vi "Pfeiffer-RVC300.ProcEvents.vi"(0 "i ref in":refnum<vi>, 5 "error in":errorcluster) -> (14 "i ref out":refnum<vi>, 19 "error out":errorcluster)   [LabVIEW 2014, in "Pfeiffer-RVC300.lvlib"]
doc: "This method is used to define the events the object will listen to. Add your own events here."
uses:
  Pfeiffer-RVC300.lvlib
  CS_Core/BaseProcess/BaseProcess.event definition.ctl
  CS_Core/CAEObj/CAEObj.event definition.ctl
  CS_Core/BaseProcess/BaseProcess.descriptor string definition.ctl
  CS_Core/BaseProcess/BaseProcess.lvlib
  CS_Core/CAEObj/CAEObj.lvlib
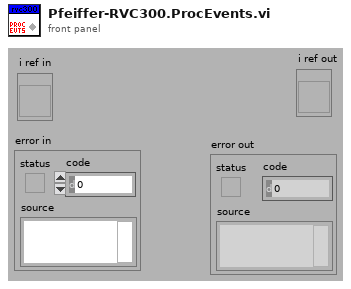
[diagram p1: front panel]
types:
  T1 = typedef "BaseProcess.lvlib/BaseProcess.event definition.ctl" = cluster{"CAEEvtDef":T2, "Data Descriptor":T3}
  T2 = typedef "CAEObj.lvlib/CAEObj.event definition.ctl" = cluster{"URL":string, "enable":bool, "ignoreResID":bool}
  T3 = typedef "BaseProcess.lvlib/BaseProcess.descriptor string definition.ctl" = string
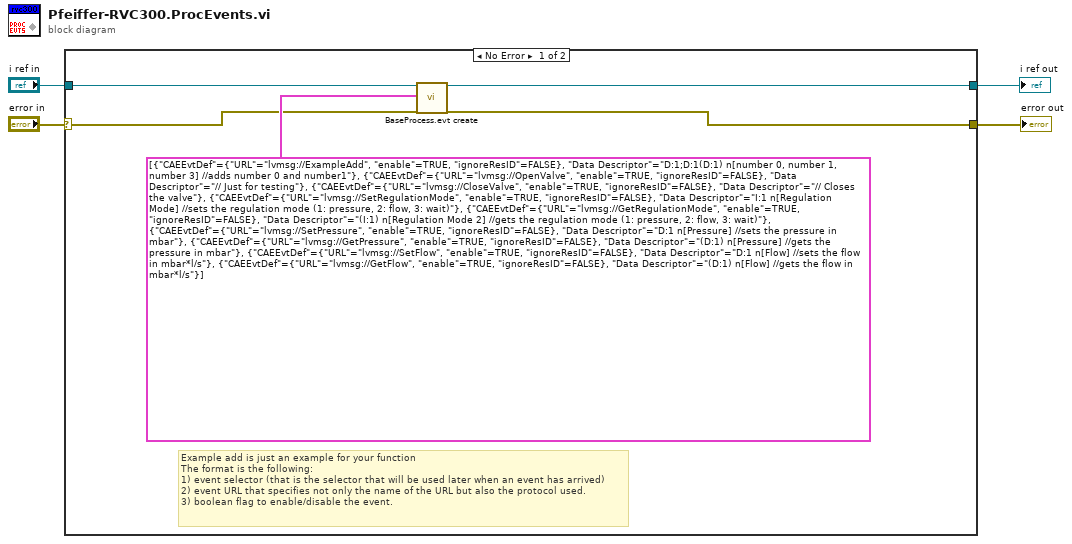
[diagram p0: block diagram]
diagram:
  n1 = case shown="No Error" "error in" {
    selector: "error in" -> [w5 w10]
    tunnel: "i ref in" -> [w9 w11]
    tunnel: [w8 w11] -> w3
    tunnel: [w7 w10] -> w2
    frame No Error {
      # "Example add is just an example for your function\nThe format is the following:\n1) event selector (that is the selector that will be used later when an event has arrived)\n2) event URL that specifies not only the name of the URL but also the protocol used.\n3) boolean flag to enable/disable the event."
      n2 = call "BaseProcess.evt create.vi"("i ref in"=w9, "newEvents"=T1[] [{"CAEEvtDef"={"URL"="lvmsg://ExampleAdd", "enable"=TRUE, "ignoreResID"=FALSE}, "Data Descriptor"="D:1;D:1(D:1) n[number 0, number 1, number 3] //adds number 0 and number1"}, {"CAEEvtDef"={"URL"="lvmsg://OpenValve", "enable"=TRUE, "ignoreResID"=FALSE}, "Data Descriptor"="// Just for testing"}, {"CAEEvtDef"={"URL"="lvmsg://CloseValve", "enable"=TRUE, "ignoreResID"=FALSE}, "Data Descriptor"="// Closes the valve"}, {"CAEEvtDef"={"URL"="lvmsg://SetRegulationMode", "enable"=TRUE, "ignoreResID"=FALSE}, "Data Descriptor"="I:1 n[Regulation Mode] //sets the regulation mode (1: pressure, 2: flow, 3: wait)"}, {"CAEEvtDef"={"URL"="lvmsg://GetRegulationMode", "enable"=TRUE, "ignoreResID"=FALSE}, "Data Descriptor"="(I:1) n[Regulation Mode 2] //gets the regulation mode (1: pressure, 2: flow, 3: wait)"}, {"CAEEvtDef"={"URL"="lvmsg://SetPressure", "enable"=TRUE, "ignoreResID"=FALSE}, "Data Descriptor"="D:1 n[Pressure] //sets the pressure in mbar"}, {"CAEEvtDef"={"URL"="lvmsg://GetPressure", "enable"=TRUE, "ignoreResID"=FALSE}, "Data Descriptor"="(D:1) n[Pressure] //gets the pressure in mbar"}, {"CAEEvtDef"={"URL"="lvmsg://SetFlow", "enable"=TRUE, "ignoreResID"=FALSE}, "Data Descriptor"="D:1 n[Flow] //sets the flow in mbar*l/s"}, {"CAEEvtDef"={"URL"="lvmsg://GetFlow", "enable"=TRUE, "ignoreResID"=FALSE}, "Data Descriptor"="(D:1) n[Flow] //gets the flow in mbar*l/s"}] ("new events"), "error in (no error)"=w5) -> ("i ref out"=w8:refnum<vi>, "error out"=w7:errorcluster)  [unwired: 13 in, 2 out]
    }
    frame Error {
    }
  }
  "i ref out" <- w3
  "error out" <- w2
